vi "Import data part 2 - csv.vi"(9 "Data filename":path) -> (2 "canceled?":bool, 3 "New Qs":T1[](array[typedef]))   [LabVIEW 2013]
uses:
  TD - Q field.ctl
  qwtblvlib/TD Quantity.ctl
  <vilib>/Utility/file.llb/Read From Spreadsheet File (string).vi
  qwtblvlib/QWTBLVLib.lvlib
panel:
  in  "Use system\ndecimal point":bool=TRUE
  out "Preview":dbl[][](array[numeric])
  in  "Skip lines:":u32
  in  "Collumn assignement":cluster{"Q name":string, "Q part":T2}[](array[cluster]) caption="Collumn assignement - To every collumn in preview assign Quantity name and type:"
  in  "Delimiter":string=","
  in  "Data in collumns":bool=TRUE
  in  "next":bool
  in  "Cancel":bool
  # "(\\t is tab)"
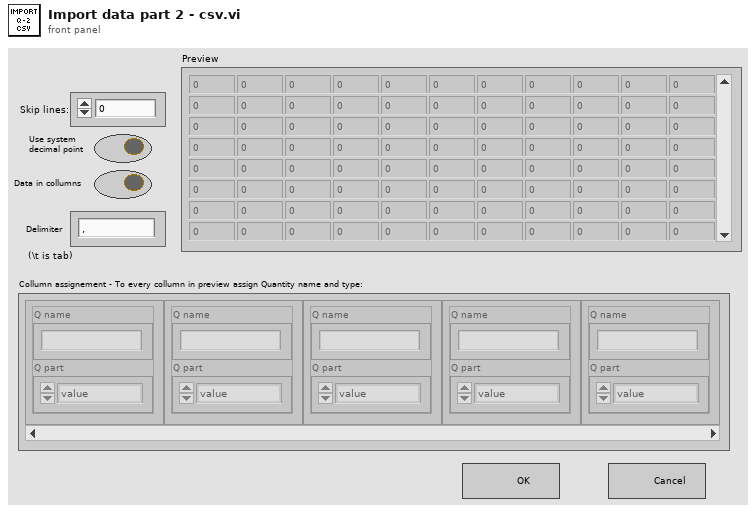
[diagram p1: front panel]
types:
  T1 = typedef "QWTBLVLib.lvlib/TD Quantity.ctl" = cluster{"Name":string, "Value":dbl[][], "Uncertainty":dbl[][], "Degrees of Freedom":dbl[][], "Correlation":dbl[][], "Randomized uncertainty":dbl[][]}
  T2 = typedef "TD - Q field.ctl" = enum16{"value", "uncertainty"}
  T3 = enum8{"Enabled", "Disabled", "Disabled and Grayed Out"}
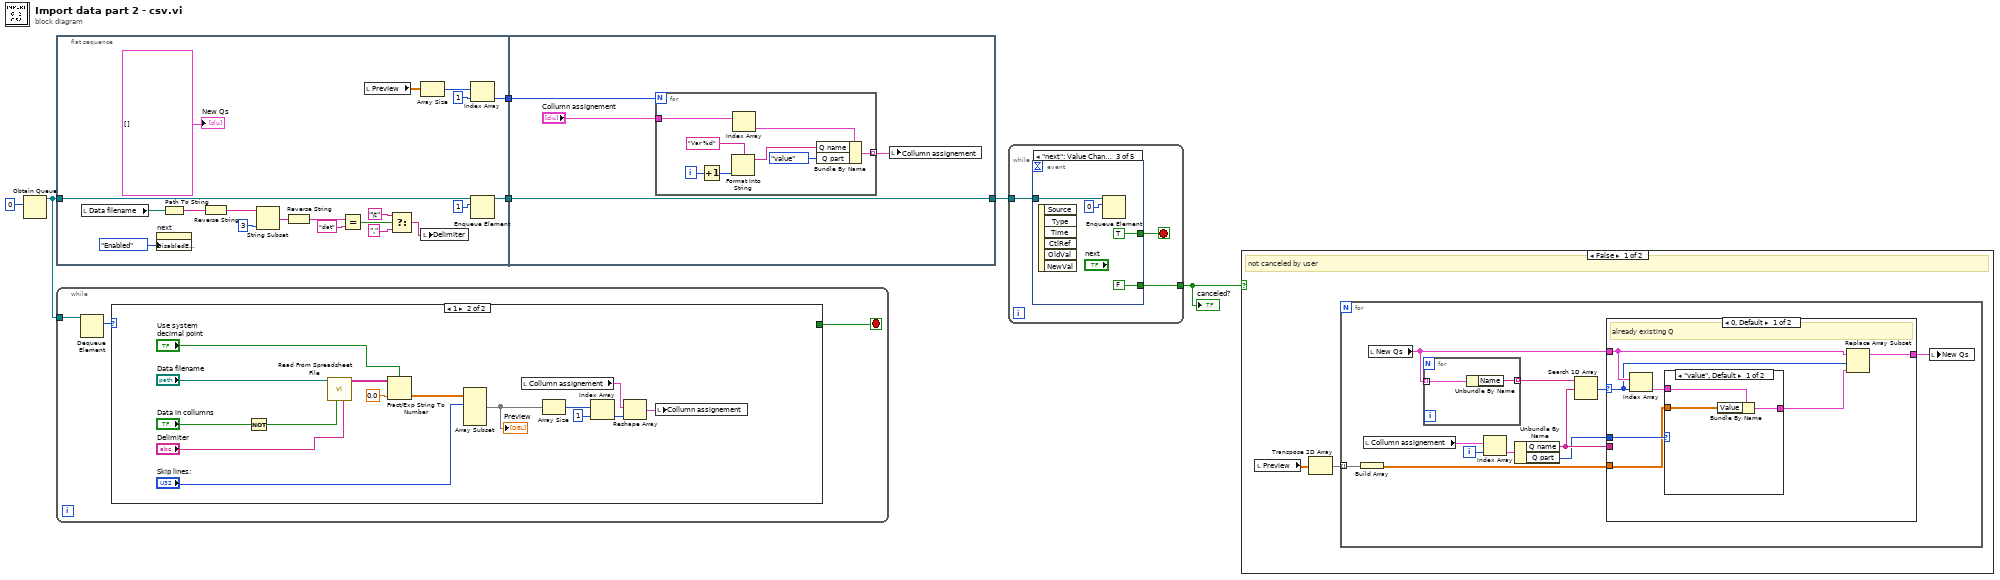
[diagram p0: block diagram]
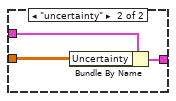
[diagram p2: hidden frame]
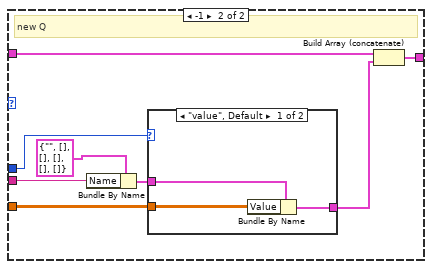
[diagram p3: hidden frame]
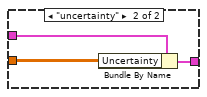
[diagram p4: hidden frame]
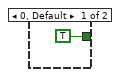
[diagram p6: hidden frame]
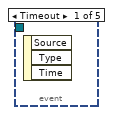
[diagram p7: hidden frame]
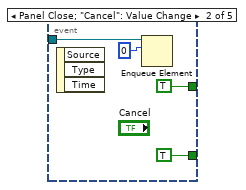
[diagram p8: hidden frame]
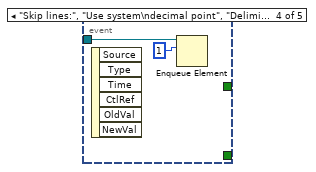
[diagram p9: hidden frame]
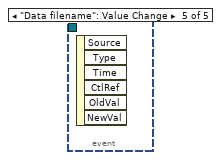
[diagram p10: hidden frame]
diagram:
  n1 = Obtain Queue(element data type=0) -> (queue out=w4:refnum<queue>)  [unwired: 4 in, 2 out]
  n2 = flat-sequence {
    tunnel: w4 -> [w25]
    tunnel: [w24] -> w3
    tunnel: [w20] -> w2
    tunnel: [w28] -> w5
    tunnel: w3 -> [w28]
    tunnel: w2 -> [w27]
    frame #0 {
      n3 = local read "Data filename"() -> (w17:path)
      n4 = property on="next" class="Bool"("DisabledEnum"=T3."Enabled" ("Disabled")) -> ()  [unwired: 2 in, 2 out]
      n5 = Path To String(path=w17) -> (string=w16:string)
      n6 = Reverse String(1:w16) -> (0:w15:string)
      n7 = String Subset(string=w15, length (rest)=3 ("length (rest)")) -> (substring=w8:string)  [unwired: 1 in]
      n8 = Reverse String(1:w8) -> (0:w7:string)
      n9 = Equal?(x=w7, y="dat") -> (x = y?=w12:bool)
      n10 = local read "Preview"() -> (w23:dbl[][])
      n11 = Select(t="\t" ("y"), s=w12, f=",") -> (s? t:f=w9:string)
      n12 = Array Size(array=w23) -> (size(s)=w22:i32[])
      n13 = local write "Delimiter"(w9) -> ()
      n14 = Index Array(array=w22, index=1) -> (element=w20:i32)
      n15 = Enqueue Element(queue=w25, element=1) -> (queue out=w24:refnum<queue>)  [unwired: 2 in, 2 out]
      "New Qs" <- T1[] [] ("New Qs")
    }
    frame #1 {
      n16 = for {
        N: w27 -> [_]
        tunnel: "Collumn assignement" -> [w38]
        tunnel: [w31] -> w29 mode=indexing
        i -> [w33]
        n17 = Increment(x=w33) -> (x+1=w34:i32)
        n18 = Format Into String(format string="Var %d", w34) -> (resulting string=w36:string)  [unwired: 2 in, 1 out]
        n19 = Index Array(array=w38) -> (element=w37:cluster{"Q name":string, "Q part":T2})  [unwired: 1 in]
        n20 = Bundle By Name(cluster=w37, "Q name"=w36, "Q part"=TD_-_Q_field."value") -> (w31:cluster{"Q name":string, "Q part":T2})
      }
      n21 = local write "Collumn assignement"(w29) -> ()
    }
  }
  n22 = while {
    tunnel: w4 -> [w41]
    stop <- w39 stop-if-true
    n23 = Dequeue Element(queue=w41) -> (element=w40:i32)  [unwired: 2 in, 3 out]
    n24 = case shown="1" w40 {
      tunnel: [TRUE _] -> w39
      frame 0, Default {
      }
      frame 1 {
        n25 = Not(x="Data in collumns") -> (.not. x?=w54:bool)
        n26 = call-poly <vilib>:"Read From Spreadsheet File.vi"("delimiter (\\t)"="Delimiter", "transpose (no:F)"=w54, "file path (dialog if empty)"="Data filename") -> ("all rows"=w57:string[][])  [unwired: 4 in, 4 out]
        n27 = Fract/Exp String To Number(use system decimal point (T)="Use system\ndecimal point", string=w57, default (0 dbl)=0.0 ("default (0 DBL)")) -> (number=w50:dbl[][])  [unwired: 1 in, 1 out]
        n28 = Array Subset(array=w50, index (row)="Skip lines:") -> (w46:dbl[][])  [unwired: 3 in]
        "Preview" <- w46
        n29 = local read "Collumn assignement"() -> (w45:cluster{"Q name":string, "Q part":T2}[])
        n30 = Array Size(array=w46) -> (size(s)=w47:i32[])
        n31 = Index Array(array=w47, index=1) -> (element=w44:i32)
        n32 = Reshape Array(w45, w44) -> (w43:cluster{"Q name":string, "Q part":T2}[])
        n33 = local write "Collumn assignement"(w43) -> ()
      }
    }
  }
  n34 = while {
    tunnel: w5 -> [w60]
    tunnel: [w58] -> w1
    stop <- w59 stop-if-true
    n35 = event shown="[2] \"next\": Value Change" {
      selector: _ -> [_ _ _ _ _]
      dyn-events: _ -> [_ _ _ _ _]
      timeout: _ -> [_ _ _ _ _]
      tunnel: [_ TRUE TRUE _ _] -> w59
      tunnel: w60 -> [_ w63 w66 w70 _]
      tunnel: [_ TRUE FALSE _ _] -> w58
      event Timeout {
        n36 = event-data() -> ()  [unwired: 1 in, 3 out]
      }
      event Panel Close; "Cancel": Value Change {
        n37 = event-data() -> ()  [unwired: 1 in, 3 out]
        n38 = Enqueue Element(queue=w63, element=0) -> ()  [unwired: 2 in, 3 out]
      }
      event "next": Value Change {
        n39 = event-data() -> ()  [unwired: 1 in, 6 out]
        n40 = Enqueue Element(queue=w66, element=0) -> ()  [unwired: 2 in, 3 out]
      }
      event "Skip lines:", "Use system\ndecimal point", "Delimiter", "Data in collumns": Value Change {
        n41 = event-data() -> ()  [unwired: 1 in, 6 out]
        n42 = Enqueue Element(queue=w70, element=1) -> ()  [unwired: 2 in, 3 out]
      }
      event "Data filename": Value Change {
        n43 = event-data() -> ()  [unwired: 1 in, 6 out]
      }
    }
  }
  "canceled?" <- w1
  n44 = case shown="False" w1 {
    frame False {
      # "not canceled by user"
      n45 = local read "Preview"() -> (w72:dbl[][])
      n46 = Transpose 2D Array(2D array=w72) -> (transposed array=w71:dbl[][])
      n47 = for {
        tunnel: w71 -> [w74] mode=indexing
        i -> [w82]
        n48 = Build Array(w74) -> (w73:dbl[][])
        n49 = local read "Collumn assignement"() -> (w83:cluster{"Q name":string, "Q part":T2}[])
        n50 = local read "New Qs"() -> (w79:T1[])
        n51 = for {
          tunnel: w79 -> [w112] mode=indexing
          tunnel: [w111] -> w81 mode=indexing
          n52 = Unbundle By Name(w112) -> ("Name"=w111:string)
        }
        n53 = Index Array(array=w83, index=w82) -> (element=w78:cluster{"Q name":string, "Q part":T2})
        n54 = Unbundle By Name(w78) -> ("Q name"=w77:string, "Q part"=w76:T2)
        n55 = Search 1D Array(1D array=w81, element=w77) -> (index of element=w80:i32)  [unwired: 1 in]
        n56 = case shown="0, Default" w80 {
          selector: w80 -> [w89 _]
          tunnel: w79 -> [w90 w99]
          tunnel: w77 -> [_ w103]
          tunnel: w76 -> [w88 w102]
          tunnel: w73 -> [w86 w100]
          tunnel: [w84 w97] -> w75
          frame 0, Default {
            # "already existing Q"
            n57 = Index Array(array=w90, index=w89) -> (element=w87:T1)
            n58 = case shown="\"value\", Default" w88 {
              tunnel: w87 -> [w93 w96]
              tunnel: w86 -> [w92 w94]
              tunnel: [w91 w95] -> w85
              frame "value", Default {
                n59 = Bundle By Name(cluster=w93, "Value"=w92) -> (w91:T1)
              }
              frame "uncertainty" {
                n60 = Bundle By Name(cluster=w96, "Uncertainty"=w94) -> (w95:T1)
              }
            }
            n61 = Replace Array Subset(array=w90, new element=w85, index=w89) -> (w84:T1[])
          }
          frame -1 {
            # "new Q"
            n62 = Bundle By Name(cluster=T1 {"Name"="", "Value"=[], "Uncertainty"=[], "Degrees of Freedom"=[], "Correlation"=[], "Randomized uncertainty"=[]} ("Q"), "Name"=w103) -> (w101:T1)
            n63 = case shown="\"value\", Default" w102 {
              tunnel: w101 -> [w107 w110]
              tunnel: w100 -> [w105 w109]
              tunnel: [w106 w108] -> w98
              frame "value", Default {
                n64 = Bundle By Name(cluster=w107, "Value"=w105) -> (w106:T1)
              }
              frame "uncertainty" {
                n65 = Bundle By Name(cluster=w110, "Uncertainty"=w109) -> (w108:T1)
              }
            }
            n66 = Build Array (concatenate)(w99, w98) -> (w97:T1[])
          }
        }
        n67 = local write "New Qs"(w75) -> ()
      }
    }
    frame True {
      # "canceled by user, no action"
    }
  }
